vi "温度采集.vi"() -> ()   [LabVIEW 2015]
uses:
  <vilib>/Utility/error.llb/DialogType.ctl
  <vilib>/DAQmx/read.llb/DAQmx Read (Analog 1D Wfm NChan NSamp).vi
  <vilib>/DAQmx/create/channels.llb/DAQmx Create Channel (AI-Voltage-Basic).vi
  <vilib>/DAQmx/configure/timing.llb/DAQmx Timing (Sample Clock).vi
  <vilib>/DAQmx/miscellaneous.llb/DAQmx Fill In Error Info.vi
  <vilib>/Analysis/2dsp.llb/1D Cross Correlation (DBL).vi
  <resource>/objmgr/daqmx.rc
  <vilib>/Analysis/NI_AALPro.lvlib
panel:
  in  "Tab Control 2":enum32{"None", "Threshold", "Levels"}(tab)=enum."Threshold"
  in  "Threshold 2":dbl=0.3400000000000002 step=0.01 format="%.2f"
  in  "Keep N Smoothest 2":i16=10 max=10
  in  "退出":bool
  out "波形图表":cluster{"[0]":dbl, "[1]":dbl}(graph)
  in  "选项卡控件":enum32{"等待", "参数设置", "采集", "信号去噪", "相关性分析"}(tab)
  in  "声音传播速度":dbl
  in  "管道压力":dbl
  in  "管道长度":dbl
  in  "管道壁厚":dbl
  in  "管道材质":string
  in  "管道直径":dbl
  in  "开始1  4":bool
  out "摄氏度 2":dbl format="%#_13g"
  out "摄氏度":dbl format="%#_13g"
  in  "采样时钟源1":tag caption="采样时钟源 1"
  in  "开始1":bool
  in  "停止1":bool
  in  "记录 2":bool
  out "记录 1":string
  in  "清空记录1":bool
  out "实际采样率 1":dbl format="%0.2f"
  in  "采样率 1":dbl=1000.0
  out "系统时间 1":string
  in  "最大值(°C)":dbl=100.0
  in  "最小值(°C)":dbl
  in  "物理通道":tag="Dev1/ai0"
  out "状态":string
  out "后置传感器":dbl[](graph)
  out "前置传感器":dbl[](graph)
  in  "文件路径 2":path
  out "末端去噪":waveform(dbl)(graph)
  out "末端原始":dynamicdata(graph)
  out "前端原始":dynamicdata(graph)
  out "前端去噪":waveform(dbl)(graph)
  in  "Tab Control":enum32{"None", "Threshold", "Levels"}(tab)=enum."Threshold"
  in  "Threshold":dbl=0.3400000000000002 step=0.01 format="%.2f"
  in  "Keep N Smoothest":i16=10 max=10
  in  "开始1  2":bool
  in  "停止1 2":bool
  in  "文件路径":path
  out "相关性时间":dbl
  out "末端信号":dynamicdata(graph)
  out "前端信号":dynamicdata(graph)
  out "波形图":waveform(dbl)(graph)
  in  "文件路径 3":path
  in  "开始1  3":bool
  in  "停止1 3":bool
  in  "传感器距离":dbl
  out "漏点位置":dbl
  # "Cut transform values below this threshold?"
  # "压力采集"
  # "Cut transform values below this threshold?"
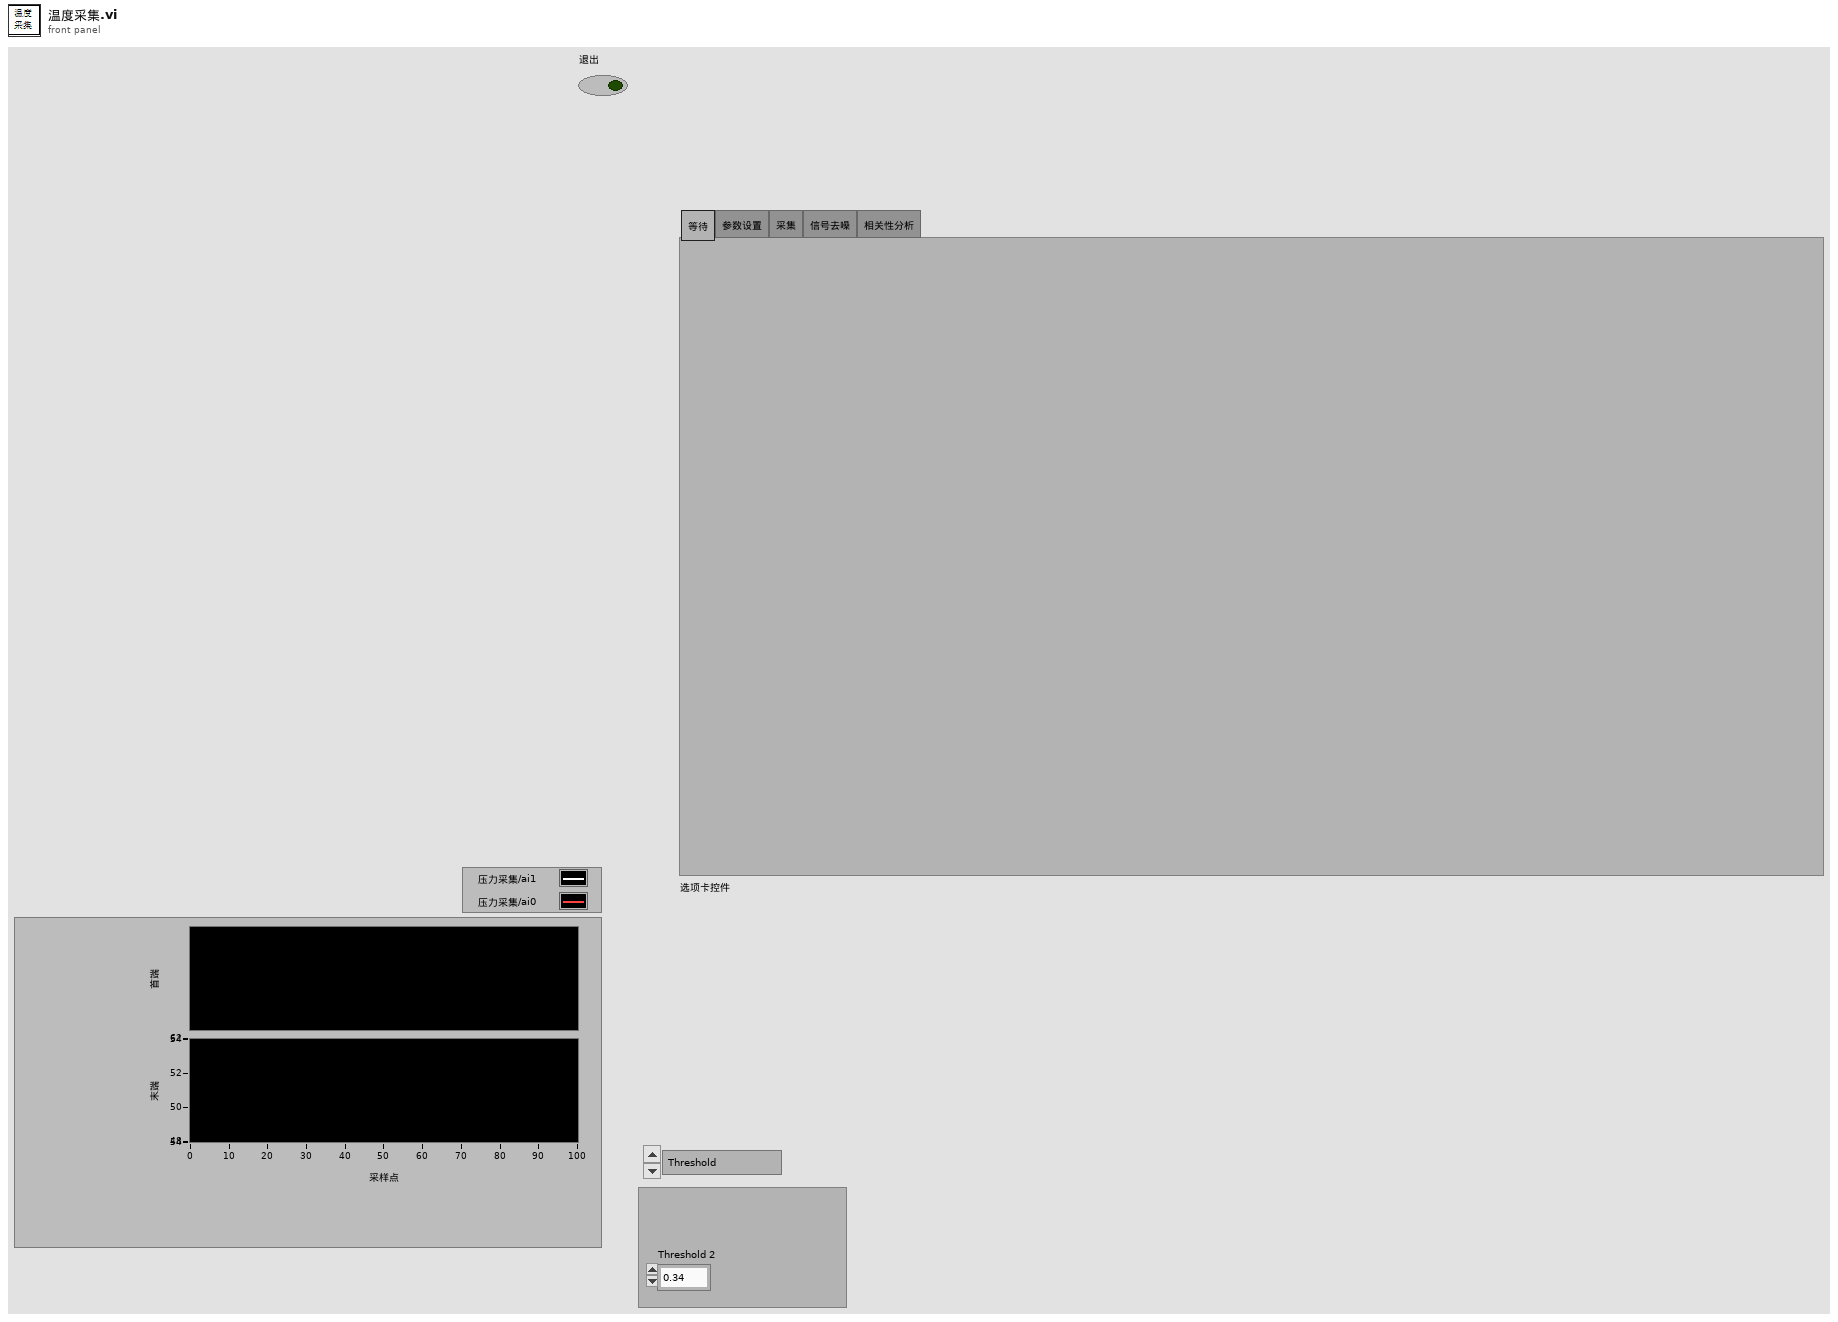
[diagram p1: front panel]
types:
  T1 = enum16{"open", "open or create", "create or replace", "create", "open (read-only)"}
  T2 = typedef "DialogType.ctl" = u16
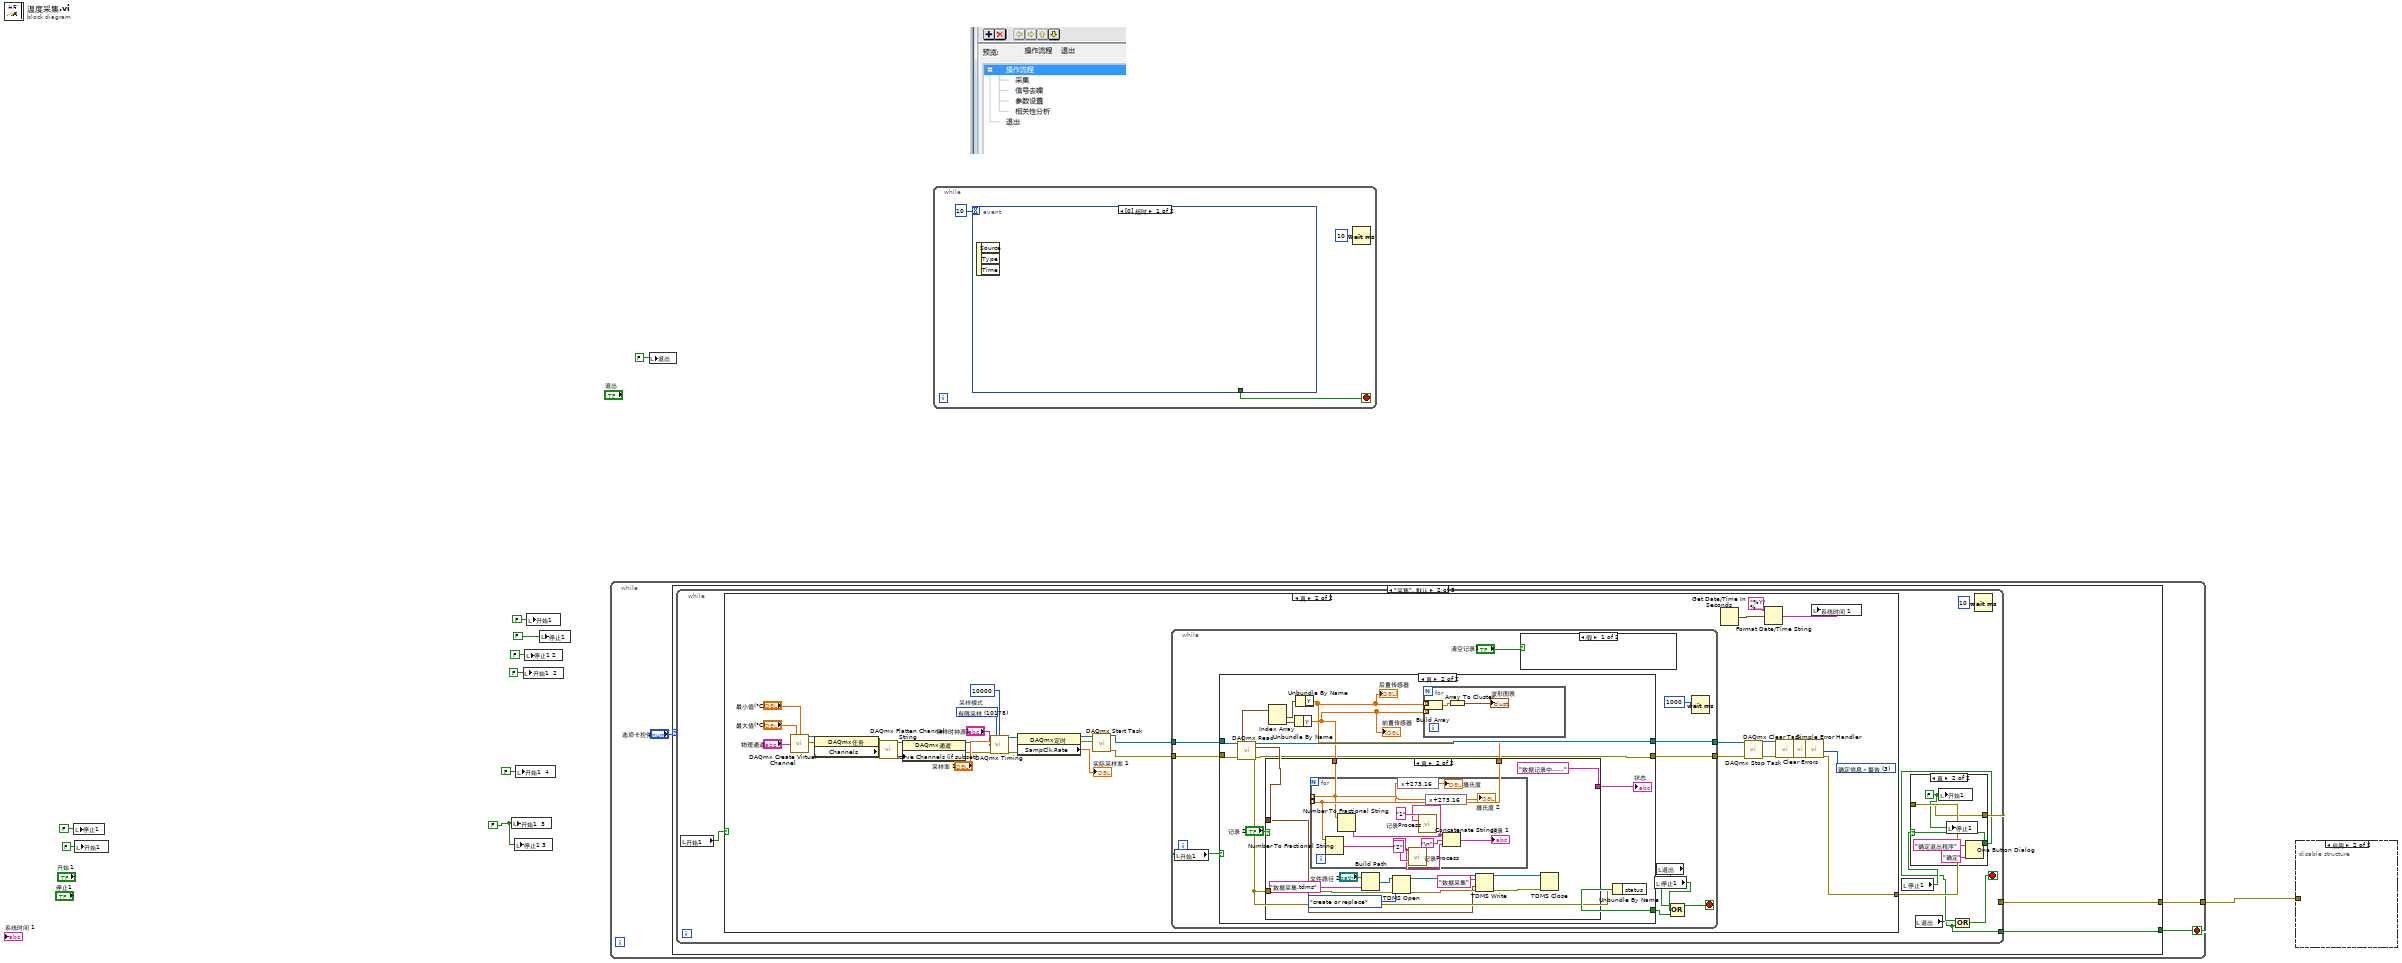
[diagram p0: block diagram]
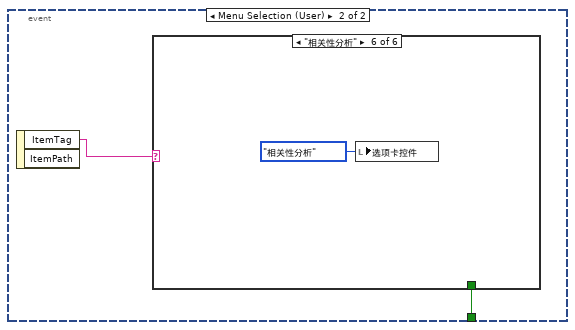
[diagram p2: hidden frame]
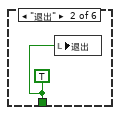
[diagram p4: hidden frame]
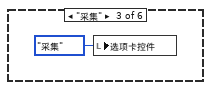
[diagram p5: hidden frame]
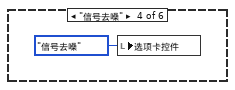
[diagram p6: hidden frame]
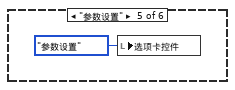
[diagram p7: hidden frame]
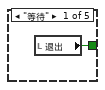
[diagram p8: hidden frame]
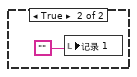
[diagram p11: hidden frame]
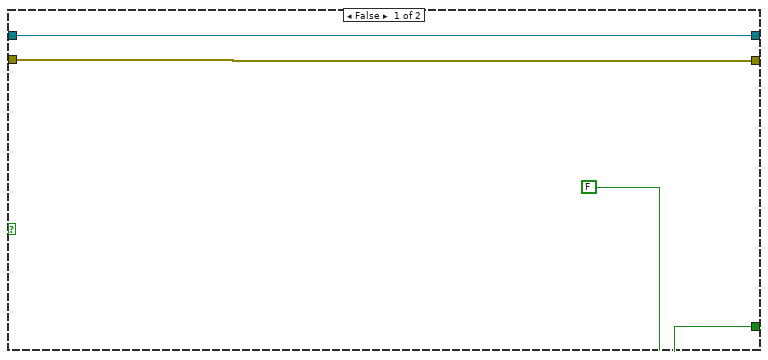
[diagram p12: hidden frame]
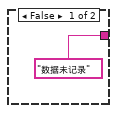
[diagram p13: hidden frame]
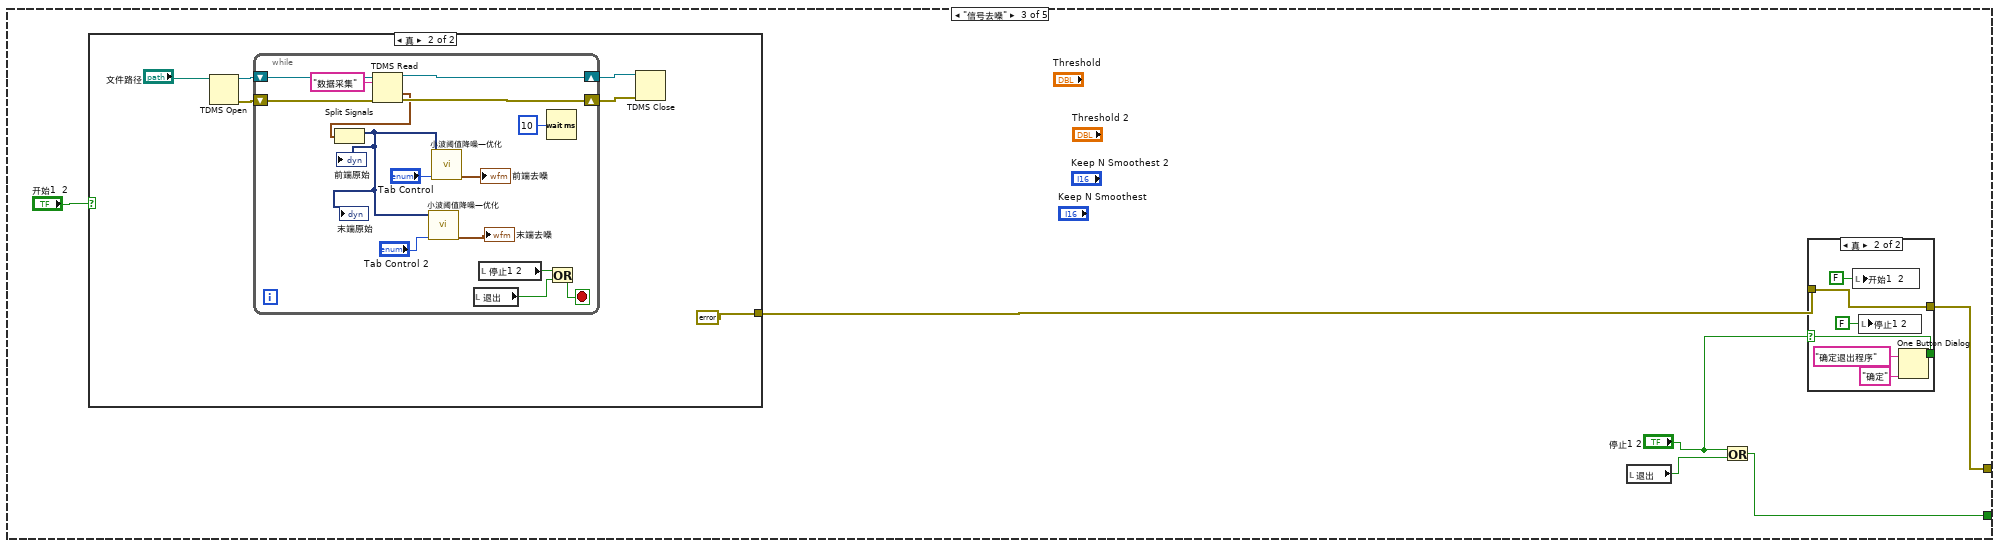
[diagram p14: hidden frame]
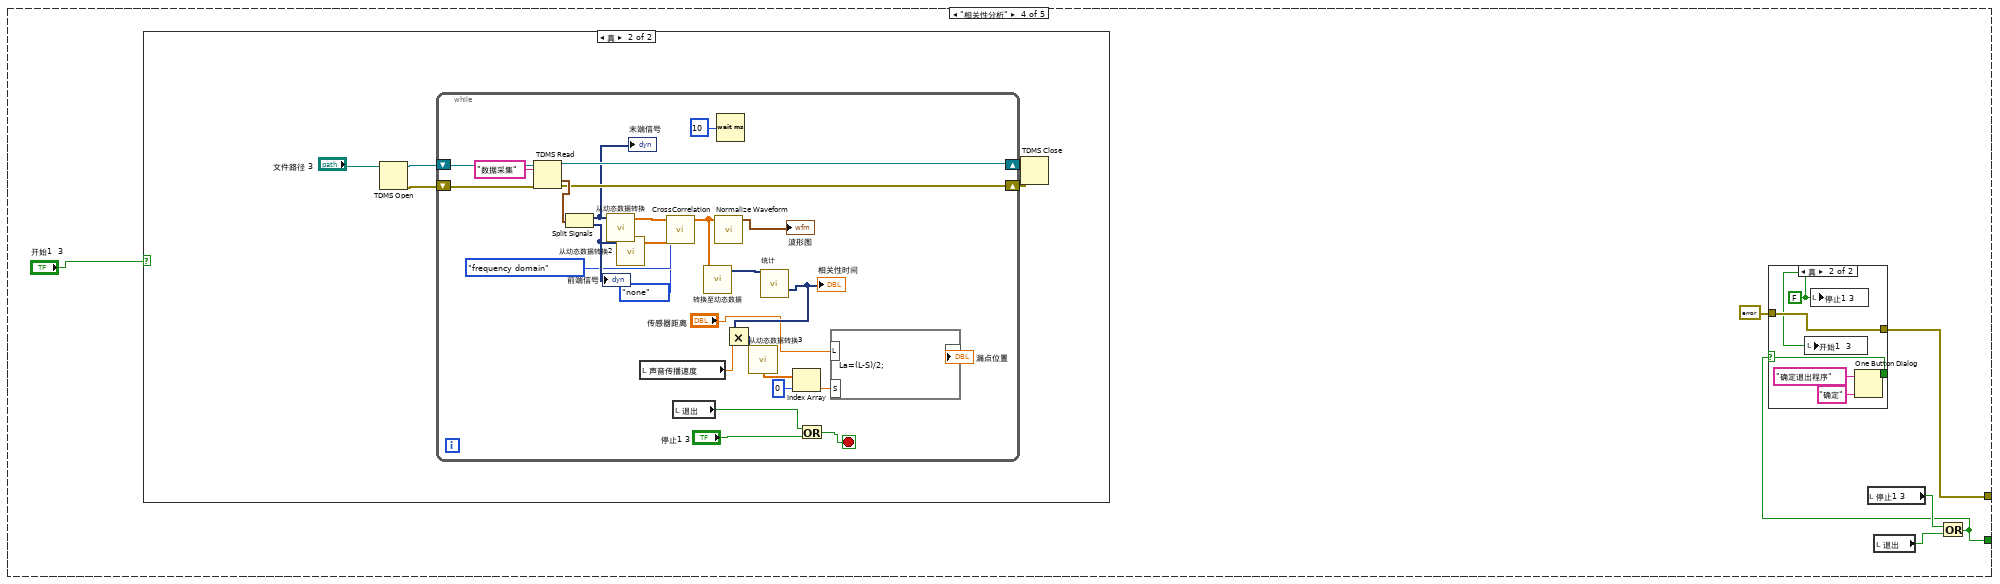
[diagram p17: hidden frame]
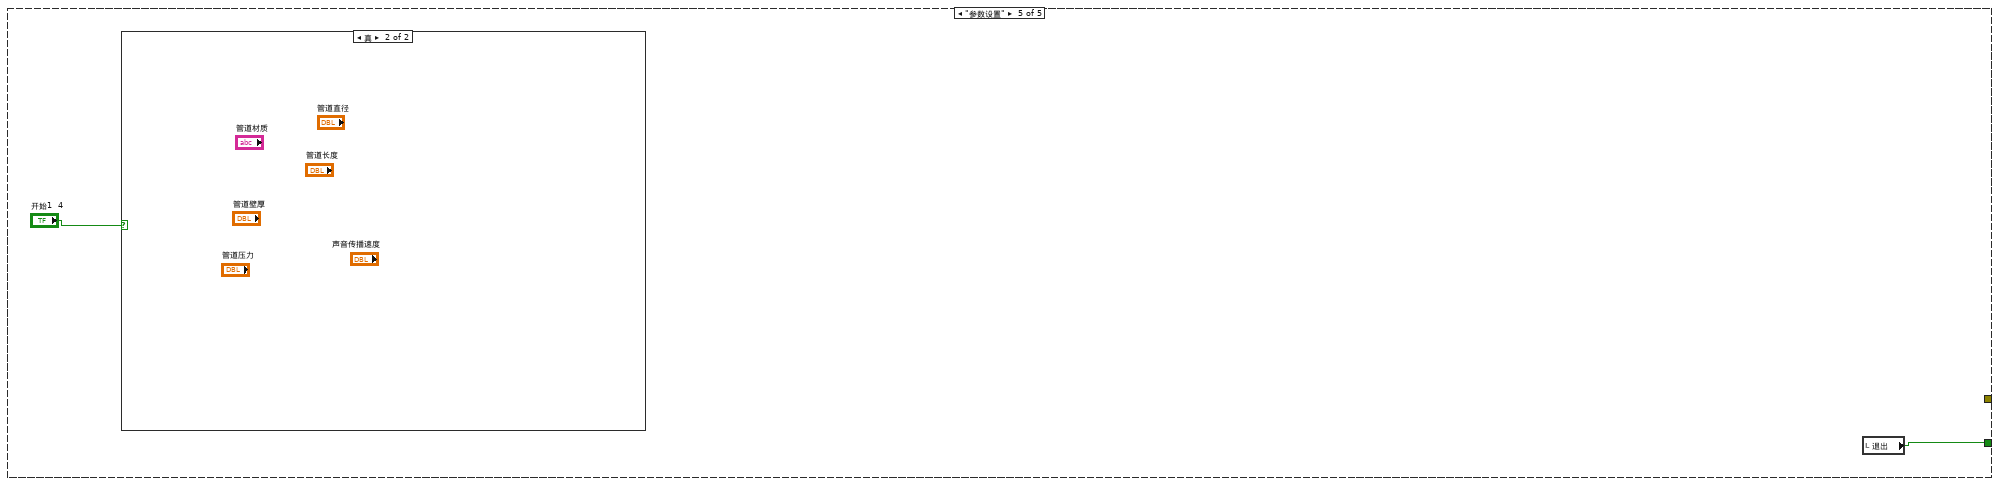
[diagram p20: hidden frame]
diagram:
  w2 = FALSE
  n1 = local write "停止1"(FALSE ("停止1")) -> ()
  n2 = local write "开始1"(FALSE ("开始1")) -> ()
  n3 = local write "开始1  3"(w2) -> ()
  n4 = local write "停止1 3"(w2) -> ()
  n5 = local write "开始1  4"(FALSE ("开始1  4")) -> ()
  n6 = local write "开始1  2"(FALSE ("开始1  2")) -> ()
  n7 = local write "停止1 2"(FALSE ("停止1 2")) -> ()
  n8 = local write "开始1"(FALSE ("开始1")) -> ()
  n9 = local write "停止1"(FALSE ("退出1")) -> ()
  n10 = while {
    tunnel: [w13] -> w8
    stop <- w11 stop-if-true
    n11 = case shown="\"采集\", 默认" "选项卡控件" {
      tunnel: [_ w16 w123 w159 _] -> w13
      tunnel: [w14 w15 w125 w158 w203] -> w11
      frame "等待" {
        n12 = local read "退出"() -> (w14:bool)
      }
      frame "采集", Default {
        n13 = while {
          tunnel: [w20] -> w16
          tunnel: [w17] -> w15
          stop <- w18 stop-if-true
          n14 = local read "开始1"() -> (w23:bool)
          n15 = case shown="真" w23 {
            tunnel: [_ w33] -> w21
            frame False {
            }
            frame True {
              w56 = 10178 items=["有限采样"=10178, "连续采样"=10123, "硬件定时单点"=12522]  # 采样模式
              w62 = T2 3 items=["无对话框", "确定信息", "继续或停止信息", "确定信息＋警告", "继续/停止＋警告"] ("对话框类型（确定信息：1）")
              n16 = call-poly <vilib>:"DAQmx Create Virtual Channel.vi"("maximum value"="最大值(°C)", "minimum value"="最小值(°C)", "physical channels"="物理通道") -> ("task out"=w54:refnum<k21>, "error out"=w53:errorcluster)  [unwired: 11 in]
              n17 = property class="DAQmx任务"(reference=w54, error in=w53) -> (reference out=w46:refnum<k21>, error out=w43:errorcluster, "Channels"=w45:refnum<k21>[])
              n18 = call <vilib>:"DAQmx Flatten Channel String.vi"("names in"=w45, "error in"=w43) -> ("names out"=w44:string, "error out"=w42:errorcluster)  [unwired: 12 in]
              n19 = property class="DAQmx通道"(reference=w46, error in=w42, "Active Channels (if subset)"=w44) -> (reference out=w52:refnum<k21>, error out=w51:errorcluster)
              n20 = call-poly <vilib>:"DAQmx Timing.vi"("task/channels in"=w52, "sample mode"=w56, "samples per channel"=10000, "rate"="采样率 1", "source"="采样时钟源1", "error in"=w51) -> ("task out"=w58:refnum<k21>, "error out"=w57:errorcluster)  [unwired: 8 in]
              n21 = property class="DAQmx定时"(reference=w58, error in=w57) -> (reference out=w49:refnum<k21>, error out=w50:errorcluster, "SampClk.Rate"=→"实际采样率 1":dbl)
              n22 = call <vilib>:"DAQmx Start Task.vi"("task/channels in"=w49, "error in"=w50) -> ("task out"=w34:refnum<k21>, "error out"=w48:errorcluster)  [unwired: 12 in]
              n23 = while "While循环" {
                tunnel: w48 -> [w71]
                tunnel: [w76] -> w60
                tunnel: w34 -> [w67]
                tunnel: [w72] -> w61
                stop <- w74 stop-if-true
                n24 = local read "开始1"() -> (w75:bool)
                n25 = case shown="真" w75 {
                  tunnel: w71 -> [w79 w92]
                  tunnel: [w79 w81] -> w76
                  tunnel: w67 -> [w80 w91]
                  tunnel: [FALSE ("status") w85] -> w73
                  tunnel: [w80 w90] -> w72
                  frame False {
                  }
                  frame True {
                    n26 = call-poly <vilib>:"DAQmx Read.vi"("task/channels in"=w91, "error in"=w92) -> ("task out"=w90:refnum<k21>, "data"=w88:waveform(dbl)[], "error out"=w81:errorcluster)  [unwired: 11 in]
                    n27 = Index Array(array=w88) -> (element #1=w87:waveform(dbl), element #2=w86:waveform(dbl))  [unwired: 2 in]
                    n28 = Unbundle By Name(w86) -> ("Y"=w82:dbl[])
                    "前置传感器" <- w82
                    n29 = Unbundle By Name(w87) -> ("Y"=w83:dbl[])
                    "后置传感器" <- w83
                    n30 = case shown="真" "记录 2" {
                      tunnel: ["数据未记录" "数据记录中……"] -> w84
                      tunnel: w88 -> [_ w99]
                      tunnel: w82 -> [_ w106]
                      tunnel: w83 -> [_ w105]
                      tunnel: w81 -> [_ w98]
                      frame False {
                      }
                      frame True {
                        n31 = for {
                          tunnel: w105 -> [w109] mode=indexing
                          tunnel: w106 -> [w110] mode=indexing
                          n32 = Number To Fractional String(number=w109) -> (F-format string=w108:string)  [unwired: 3 in]
                          n33 = Number To Fractional String(number=w110) -> (F-format string=w111:string)  [unwired: 3 in]
                          n34 = expression code="x+273.16"(w109) -> (→"摄氏度":dbl)
                          n35 = call "记录Process.vi"("采集通道"="2", "记录"=w108) -> ()  [unwired: 9 in, 1 out]
                          n36 = call "记录Process.vi"("采集通道"="1", "记录"=w111) -> ()  [unwired: 9 in, 1 out]
                          n37 = expression code="x+273.16"(w110) -> (→"摄氏度 2":dbl)
                          n38 = Concatenate Strings(w111, "\n", w108) -> (→"记录 1":string)
                        }
                        n39 = Build Path(base path="文件路径 2", name or relative path="数据采集.tdms" ("名称或相对路径")) -> (appended path=w94:path)
                        n40 = TDMS Open(8:w98, 10:T1."create or replace" ("操作(0:open)"), 11:w94) -> (0:w103:errorcluster, 3:w104:refnum<k34>)  [unwired: 4 in]
                        n41 = TDMS Write(0:w104, 5:"数据采集" ("组名称输入（无标题）"), 9:w99, 11:w103) -> (4:w101:refnum<k34>, 15:w102:errorcluster)  [unwired: 2 in, 2 out]
                        n42 = TDMS Close(8:w102, 11:w101) -> ()  [unwired: 2 out]
                      }
                    }
                    "状态" <- w84
                    n43 = for {
                      tunnel: w83 -> [w121] mode=indexing
                      tunnel: w82 -> [w120] mode=indexing
                      n44 = Build Array(w121, w120) -> (w119:dbl[])
                      n45 = Array To Cluster(array=w119) -> (cluster=→"波形图表":cluster{"[0]":dbl, "[1]":dbl})
                    }
                    n46 = Unbundle By Name(w81) -> ("status"=w85:bool)
                  }
                }
                n47 = case shown="假" "清空记录1" {
                  frame False {
                  }
                  frame True {
                    n48 = local write "记录 1"("") -> ()
                  }
                }
                n49 = local read "停止1"() -> (w70:bool)
                n50 = local read "退出"() -> (w66:bool)
                n51 = Compound Arithmetic op=OR ("复合运算")(w66, w70, w73) -> (w74:bool)
                n52 = Wait (ms)(milliseconds to wait=u32 1000 ("等待时间（毫秒）")) -> ()  [unwired: 1 out]
              }
              n53 = Get Date/Time In Seconds() -> (seconds since 1Jan1904=w35:timestamp)
              n54 = call <vilib>:"DAQmx Stop Task.vi"("task/channels in"=w61, "error in"=w60) -> ("task out"=w64:refnum<k21>, "error out"=w63:errorcluster)  [unwired: 12 in]
              n55 = Format Date/Time String(time format string (%c)="%Y/%m/%d %H:%M:%S" ("时间格式字符串(%c)"), seconds (now)=w35) -> (date/time string=w36:string)  [unwired: 1 in]
              n56 = call <vilib>:"DAQmx Clear Task.vi"("task in"=w64, "error in"=w63) -> ("error out"=w65:errorcluster)  [unwired: 13 in]
              n57 = call <vilib>:"Clear Errors.vi"("error in (no error)"=w65) -> ("error out"=w32:errorcluster)  [unwired: 5 in, 1 out]
              n58 = call <vilib>:"Simple Error Handler.vi"("type of dialog (OK msg:1)"=w62, "error in (no error)"=w32) -> ("error out"=w33:errorcluster)  [unwired: 3 in, 4 out]
              n59 = local write "系统时间 1"(w36) -> ()
            }
          }
          n60 = local read "停止1"() -> (w22:bool)
          n61 = case shown="真" w22 {
            selector: w22 -> [w26 w30]
            tunnel: w21 -> [w25 w31]
            tunnel: [w25 w31] -> w20
            tunnel: [w26 w30] -> w19
            frame False {
            }
            frame True {
              w27 = FALSE ("开始1")
              n62 = local write "开始1"(w27) -> ()
              n63 = local write "停止1"(w27) -> ()
              n64 = One Button Dialog(message="确定退出程序" ("消息"), button name ("OK")="确定" ("按钮名称（“确定”）")) -> ()  [unwired: 1 out]
            }
          }
          n65 = local read "退出"() -> (w17:bool)
          n66 = Compound Arithmetic op=OR ("复合运算")(w19, w17) -> (w18:bool)
          n67 = Wait (ms)(milliseconds to wait=u32 10 ("等待时间（毫秒）")) -> ()  [unwired: 1 out]
        }
      }
      frame "信号去噪" {
        n68 = case shown="真" "开始1  2" {
          tunnel: [_ errorcluster {"status"=FALSE, "code"=0, "source"=""} ("错误常量")] -> w122
          frame False {
          }
          frame True {
            n69 = TDMS Open(11:"文件路径") -> (0:w137:errorcluster, 3:w136:refnum<k34>)  [unwired: 6 in]
            n70 = while {
              shift-right: [w151] -> w138
              shift-left: w137 -> [w150]
              shift-right: [w152] -> w139
              shift-left: w136 -> [w149]
              stop <- w142 stop-if-true
              n71 = TDMS Read(0:w149, 5:"数据采集" ("组名称输入"), 11:w150) -> (4:w152:refnum<k34>, 10:w147:waveform(dbl)[], 15:w151:errorcluster)  [unwired: 5 in, 3 out]
              n72 = Split Signals(w147) -> (w146:dynamicdata)  [unwired: 2 in, 1 out]
              "前端原始" <- w146
              "末端原始" <- w146
              n73 = call "小波阈值降噪—优化.vi"("Tab Control"="Tab Control 2", "signal out"=w146) -> ("Denoised Signal"=→"末端去噪":waveform(dbl))  [unwired: 4 in, 2 out]
              n74 = call "小波阈值降噪—优化.vi"("Tab Control"="Tab Control", "signal out"=w146) -> ("Denoised Signal"=→"前端去噪":waveform(dbl))  [unwired: 4 in, 2 out]
              n75 = local read "退出"() -> (w143:bool)
              n76 = local read "停止1 2"() -> (w144:bool)
              n77 = Wait (ms)(milliseconds to wait=u32 10 ("等待时间（毫秒）")) -> ()  [unwired: 1 out]
              n78 = Or(x=w144, y=w143) -> (x .or. y?=w142:bool)
            }
            n79 = TDMS Close(8:w138, 11:w139) -> ()  [unwired: 2 out]
          }
        }
        n80 = local read "退出"() -> (w126:bool)
        n81 = Or(x="停止1 2", y=w126) -> (x .or. y?=w125:bool)
        n82 = case shown="真" "停止1 2" {
          selector: "停止1 2" -> [w129 w134]
          tunnel: w122 -> [w128 w135]
          tunnel: [w128 w135] -> w123
          tunnel: [w129 w134] -> _
          frame False {
          }
          frame True {
            n83 = local write "开始1  2"(FALSE ("开始1  2")) -> ()
            n84 = local write "停止1 2"(FALSE ("停止1 2")) -> ()
            n85 = One Button Dialog(message="确定退出程序" ("消息"), button name ("OK")="确定" ("按钮名称（“确定”）")) -> ()  [unwired: 1 out]
          }
        }
      }
      frame "相关性分析" {
        n86 = case shown="真" "开始1  3" {
          frame False {
          }
          frame True {
            n87 = TDMS Open(11:"文件路径 3") -> (0:w172:errorcluster, 3:w173:refnum<k34>)  [unwired: 6 in]
            n88 = while {
              shift-right: [w196] -> w171
              shift-left: w173 -> [w198]
              shift-right: [w195] -> w170
              shift-left: w172 -> [w197]
              stop <- w192 stop-if-true
              n89 = TDMS Read(0:w198, 5:"数据采集" ("组名称输入"), 11:w197) -> (4:w196:refnum<k34>, 10:w200:waveform(dbl)[], 15:w195:errorcluster)  [unwired: 5 in, 3 out]
              n90 = Split Signals(w200) -> (w194:dynamicdata, w193:dynamicdata)  [unwired: 2 in]
              "末端信号" <- w194
              "前端信号" <- w193
              n91 = call "从动态数据转换"("Dynamic Data Type"=w194) -> ("Array"=w189:dbl[])  [unwired: 3 in]
              n92 = call "从动态数据转换2"("Dynamic Data Type"=w193) -> ("Array"=w188:dbl[])  [unwired: 3 in]
              n93 = local read "声音传播速度"() -> (w182:dbl)
              n94 = call-poly <vilib>:"CrossCorrelation.vi"("normalization"=enum32{"none", "unbiased", "biased"}."none", "algorithm"=enum32{"direct", "frequency domain"}."frequency domain", "Y"=w188, "X"=w189) -> ("Rxy"=w185:dbl[])  [unwired: 6 in, 1 out]
              n95 = local read "退出"() -> (w191:bool)
              n96 = call "转换至动态数据"("Array"=w185) -> ("Dynamic Data Type"=w183:dynamicdata)  [unwired: 3 in]
              n97 = call <vilib>:"Normalize Waveform.vi"("waveform in"=w185) -> ("normalized waveform"=→"波形图":waveform(dbl))  [unwired: 7 in, 3 out]
              n98 = Wait (ms)(milliseconds to wait=u32 10 ("等待时间（毫秒）")) -> ()  [unwired: 1 out]
              n99 = call "统计"("Signals"=w183) -> ("Time of Maximum"=w181:dynamicdata)  [unwired: 25 in, 1 out]
              "相关性时间" <- w181
              n100 = Multiply(x=w181, y=w182) -> (x*y=w180:dynamicdata)
              n101 = call "从动态数据转换3"("Dynamic Data Type"=w180) -> ("Array"=w179:dbl[])  [unwired: 3 in]
              n102 = Index Array(array=w179, index=0 ("索引")) -> (element=w176:dbl)
              n103 = Or(x=w191, y="停止1 3") -> (x .or. y?=w192:bool)
              n104 = formula code="La=(L-S)/2;"("L"="传感器距离", "S"=w176) -> ("La"=→"漏点位置":dbl)
            }
            n105 = TDMS Close(8:w170, 11:w171) -> ()  [unwired: 2 out]
          }
        }
        n106 = local read "停止1 3"() -> (w160:bool)
        n107 = local read "退出"() -> (w161:bool)
        n108 = Or(x=w160, y=w161) -> (x .or. y?=w158:bool)
        n109 = case shown="真" w158 {
          selector: w158 -> [w164 w168]
          tunnel: errorcluster {"status"=FALSE, "code"=0, "source"=""} ("error out") -> [w163 w169]
          tunnel: [w163 w169] -> w159
          tunnel: [w164 w168] -> _
          frame False {
          }
          frame True {
            w165 = FALSE ("停止1 3")
            n110 = local write "开始1  3"(w165) -> ()
            n111 = local write "停止1 3"(w165) -> ()
            n112 = One Button Dialog(message="确定退出程序" ("消息"), button name ("OK")="确定" ("按钮名称（“确定”）")) -> ()  [unwired: 1 out]
          }
        }
      }
      frame "参数设置" {
        n113 = case shown="真" "开始1  4" {
          frame False {
          }
          frame True {
          }
        }
        n114 = local read "退出"() -> (w203:bool)
      }
    }
  }
  n115 = local write "退出"(FALSE ("退出")) -> ()
  n116 = while {
    stop <- w204 stop-if-true
    n117 = event shown="[0] 超时" {
      selector: _ -> [_ _]
      dyn-events: _ -> [_ _]
      timeout: 10 -> [_ _]
      tunnel: [_ w207] -> w204
      event Timeout {
        n118 = event-data() -> ()  [unwired: 1 in, 3 out]
      }
      event Menu Selection (User) {
        n119 = event-data() -> ("ItemTag"=w208:string)  [unwired: 1 in, 1 out]
        n120 = case shown="\"相关性分析\"" w208 {
          tunnel: [_ w209 _ _ _ _] -> w207
          frame "假", Default {
          }
          frame "退出" {
            w209 = TRUE
            n121 = local write "退出"(w209) -> ()
          }
          frame "采集" {
            n122 = local write "选项卡控件"(enum32{"等待", "参数设置", "采集", "信号去噪", "相关性分析"}."采集" ("选项卡控件")) -> ()
          }
          frame "信号去噪" {
            n123 = local write "选项卡控件"(enum32{"等待", "参数设置", "采集", "信号去噪", "相关性分析"}."信号去噪" ("选项卡控件")) -> ()
          }
          frame "参数设置" {
            n124 = local write "选项卡控件"(enum32{"等待", "参数设置", "采集", "信号去噪", "相关性分析"}."参数设置" ("选项卡控件")) -> ()
          }
          frame "相关性分析" {
            n125 = local write "选项卡控件"(enum32{"等待", "参数设置", "采集", "信号去噪", "相关性分析"}."相关性分析" ("选项卡控件")) -> ()
          }
        }
      }
    }
    n126 = Wait (ms)(milliseconds to wait=u32 10 ("等待时间（毫秒）")) -> ()  [unwired: 1 out]
  }
  n127 = disable-structure shown="启用" {
    disable-tunnel: w8 -> [w214 _]
    frame Disabled {
      n128 = control-ref of="本VI"() -> (w215:refnum<vi>)
      n129 = invoke class="VI" method="FP.Close"(reference=w215, error in=w214) -> ()  [unwired: 1 in, 3 out]
    }
    frame Enabled {
    }
  }
